vi "RTS Delete Key Config File.vi"(8 "error in (no error)":errorcluster, 11 "Refnum in":T1) -> (0 "error out":errorcluster, 3 "Refnum out":T1)   [LabVIEW 2016]
uses:
  <vilib>/Utility/config.llb/Config Data RefNum.ctl
  <vilib>/Utility/config.llb/NI_LVConfig.lvlib
panel:
  out "key names":string[][](array[string])
  out "section names":string[](array[string])
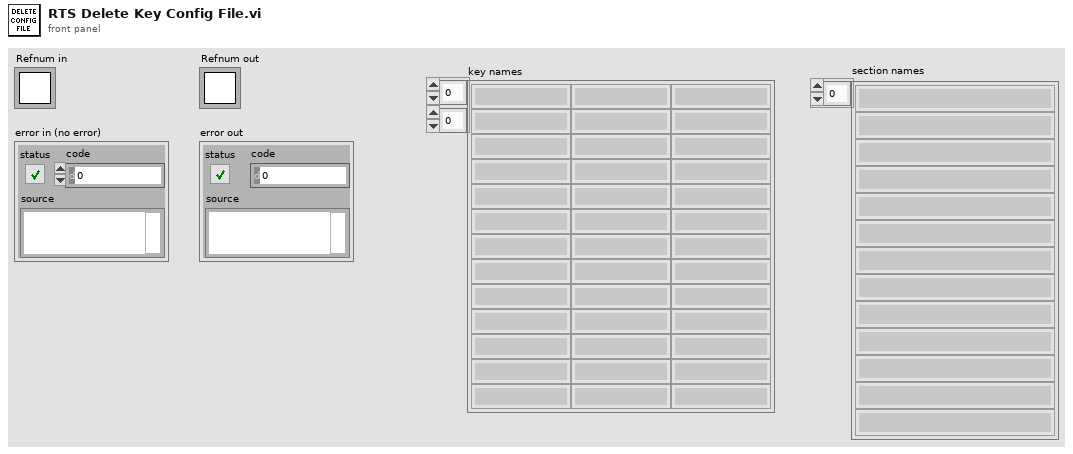
[diagram p1: front panel]
types:
  T1 = typedef "NI_LVConfig.lvlib/Config Data RefNum.ctl" = refnum<k1>
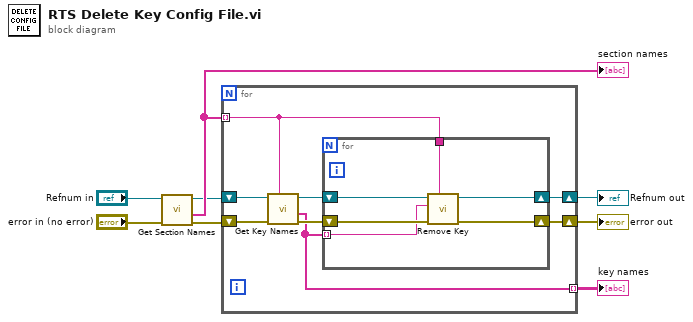
[diagram p0: block diagram]
diagram:
  n1 = call <vilib>:"Get Section Names.vi"("error in (no error)"="error in (no error)", "refnum"="Refnum in") -> ("error out"=w2:errorcluster, "section names"=w6:string[], "refnum out"=w3:T1)  [unwired: 7 in]
  "section names" <- w6
  n2 = for {
    shift-right: [w16] -> w4
    shift-left: w2 -> [w14]
    shift-right: [w15] -> w5
    shift-left: w3 -> [w13]
    tunnel: w6 -> [w10] mode=indexing
    tunnel: [w9] -> w1 mode=indexing
    n3 = call <vilib>:"Get Key Names.vi"("section"=w10, "error in (no error)"=w14, "refnum"=w13) -> ("error out"=w12:errorcluster, "key names"=w9:string[], "refnum out"=w11:T1)  [unwired: 5 in, 1 out]
    n4 = for {
      tunnel: w10 -> [w18]
      shift-right: [w22] -> w16
      shift-left: w12 -> [w20]
      shift-right: [w21] -> w15
      shift-left: w11 -> [w19]
      tunnel: w9 -> [w17] mode=indexing
      n5 = call <vilib>:"Remove Key.vi"("section"=w18, "error in (no error)"=w20, "key"=w17, "refnum"=w19) -> ("error out"=w22:errorcluster, "refnum out"=w21:T1)  [unwired: 5 in, 1 out]
    }
  }
  "Refnum out" <- w5
  "error out" <- w4
  "key names" <- w1
